vi "常规五参数测量数据区.vi"(11 "数组":u16[](array[numeric]) format="%04xH") -> (3 "测量数据区":T1)   [LabVIEW 2016, in "斯坦道仪器.lvlib"]
panel:
  # "共占用28 WORD"
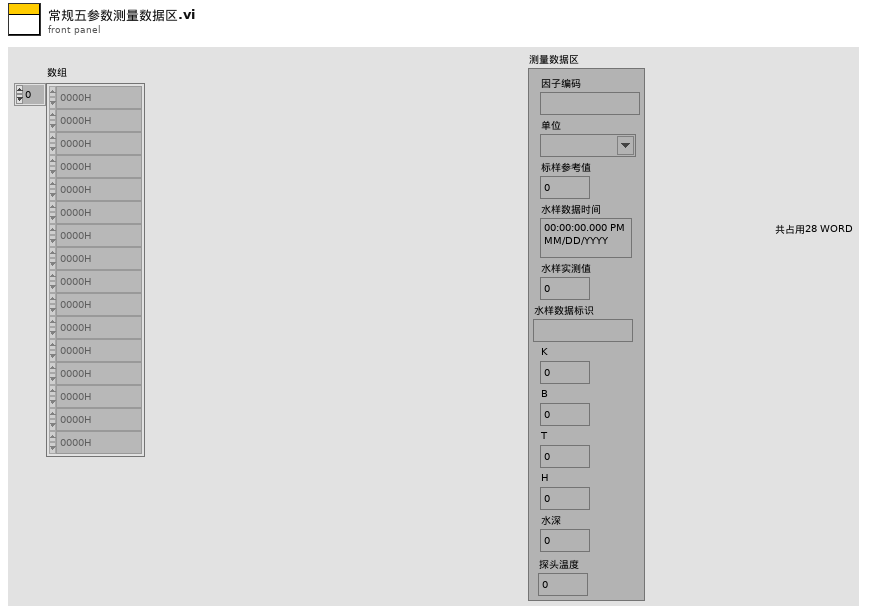
[diagram p1: front panel]
types:
  T1 = cluster{"因子编码":string, "单位":string, "标样参考值":sgl, "水样数据时间":timestamp, "水样实测值":sgl, "水样数据标识":string, "K":sgl, "B":sgl, "T":sgl, "H":sgl, "水深":sgl, "探头温度":sgl}
  T2 = cluster{string, string, "FLOAT":sgl, "time stamp":timestamp, "数值":sgl, "string":string, "FLOAT":sgl, "FLOAT":sgl, "FLOAT":sgl, "FLOAT":sgl, "FLOAT":sgl, "FLOAT":sgl}
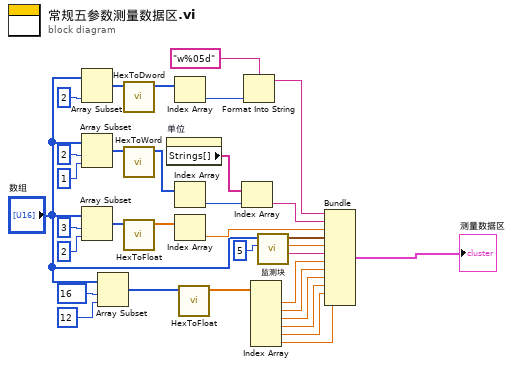
[diagram p0: block diagram]
diagram:
  n1 = Array Subset(array="数组", length=2 ("长度")) -> (w34:u16[])  [unwired: 1 in]
  n2 = Array Subset(array="数组", index=2 ("索引"), length=1 ("长度")) -> (w29:u16[])
  n3 = Array Subset(array="数组", index=3 ("索引"), length=2 ("长度")) -> (w25:u16[])
  n4 = Array Subset(array="数组", index=16 ("索引"), length=12 ("长度")) -> (w15:u16[])
  n5 = call "HexToDword.vi"("数组"=w34) -> ("DWORD"=w32:i32[])  [unwired: 10 in]
  n6 = call "HexToWord.vi"("数组"=w29) -> ("WORD"=w28:u16[])  [unwired: 10 in]
  n7 = call "HexToFloat.vi"("数组"=w25) -> ("FLOAT"=w24:sgl[])  [unwired: 10 in]
  n8 = property on="单位" class="CmbBox"() -> ("Strings[]"=w5:string[])  [unwired: 2 in, 2 out]
  n9 = Index Array(array=w32) -> (element=w3:i32)  [unwired: 1 in]
  n10 = Index Array(array=w28) -> (element=w7:u16)  [unwired: 1 in]
  n11 = Index Array(array=w24) -> (element=w23:sgl)  [unwired: 1 in]
  n12 = call "HexToFloat.vi"("数组"=w15) -> ("FLOAT"=w14:sgl[])  [unwired: 10 in]
  n13 = Index Array(array=w5, index=w7) -> (element=w6:string)
  n14 = Format Into String(format string="w%05d" ("格式字符串"), w3) -> (resulting string=w2:string)  [unwired: 2 in, 1 out]
  n15 = Index Array(array=w14) -> (element #1=w13:sgl, element #2=w12:sgl, element #3=w11:sgl, element #4=w10:sgl, element #5=w9:sgl, element #6=w1:sgl)  [unwired: 6 in]
  n16 = call "监测块.vi"("索引"=5, "数组"="数组") -> ("string"=w20:string, "数值"=w21:sgl, "time stamp"=w22:timestamp)  [unwired: 7 in]
  n17 = Bundle(w2, w6, "FLOAT"=w23, "time stamp"=w22, "数值"=w21, "string"=w20, "FLOAT"=w13, "FLOAT"=w12, "FLOAT"=w11, "FLOAT"=w10, "FLOAT"=w9, "FLOAT"=w1) -> (→"测量数据区":T2)  [unwired: 1 in]
